vi "to_json.vi"(8 "error in":errorcluster, 11 "mcap in":refnum<class "mcap.lvclass">) -> (0 "error out":errorcluster, 2 "json":string, 3 "mcap out":refnum<class "mcap.lvclass">)   [LabVIEW 2020, in "nominal types.lvlib" / "timestampManifest.lvlib" / "mcap.lvclass"]
uses:
  mcap.lvclass
  mcap.lvclass/mcap.ctl
  <vilib>/JDP Science/JSONtext/JSONtext.lvlib
  include/include.lvclass
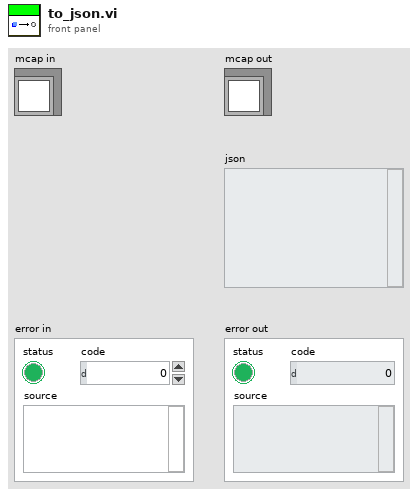
[diagram p1: front panel]
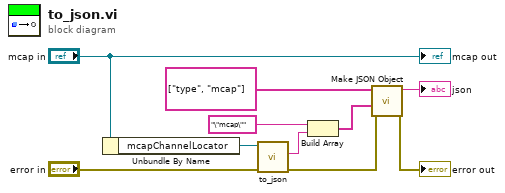
[diagram p0: block diagram]
diagram:
  n1 = Unbundle By Name("mcap in") -> ("mcapChannelLocator"=w9:refnum<class "include.lvclass">)
  n2 = call-dynamic "to_json.vi"("error in"="error in", "include in"=w9) -> ("error out"=w2:errorcluster, "json"=w7:string)  [unwired: 7 in, 1 out]
  n3 = Build Array("\"mcap\"" ("element"), w7) -> (w4:string[])
  n4 = call <vilib>:"Make JSON Object.vi"("error in (no error)"=w2, "JSON Items"=w4, "Item Names"=string[] ["type", "mcap"]) -> ("error out"=→"error out":errorcluster, "<JSON>"=→"json":string)  [unwired: 7 in]
  "mcap out" <- "mcap in"
